vi "Set Panel Size.vi"(10 "Boolean":bool, 11 "VI in":refnum<vi>) -> (0 "error out":errorcluster)   [LabVIEW 2019, in "Panther Dashboard.lvlib"]
uses:
  Panther Dashboard.lvlib
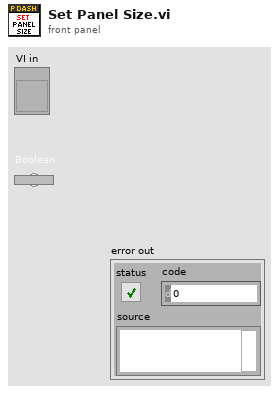
[diagram p1: front panel]
types:
  T1 = typedef "LVRectTypeDef.ctl" = cluster{"Left":i16, "Top":i16, "Right":i16, "Bottom":i16}
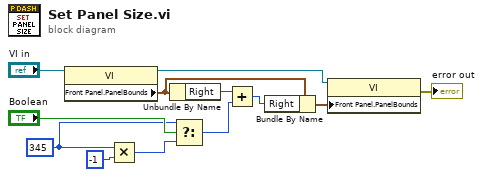
[diagram p0: block diagram]
diagram:
  w3 = i16 345 ("Splitter Position")
  n1 = property class="VI"(reference="VI in") -> (reference out=w11:refnum<vi>, "Front Panel.PanelBounds"=w7:T1)  [unwired: 1 in, 1 out]
  n2 = Multiply(x=w3, y=i16 -1) -> (x*y=w1:i16)
  n3 = Unbundle By Name(w7) -> ("Right"=w6:i16)
  n4 = Select(t=w3, s="Boolean", f=w1) -> (s? t:f=w4:i16)
  n5 = Add(x=w6, y=w4) -> (x+y=w5:i16)
  n6 = Bundle By Name(cluster=w7, "Right"=w5) -> (w8:T1)
  n7 = property class="VI"(reference=w11, "Front Panel.PanelBounds"=w8) -> (error out=→"error out":errorcluster)  [unwired: 1 in, 1 out]
